vi "get.Bytes.vi"(8 "error in (no error)":errorcluster, 11 "SequencedUnitHeader in":refnum<class "SequencedUnitHeader.lvclass">) -> (0 "error out":errorcluster, 2 "Bytes.Out":u8[](array[numeric]), 3 "SequencedUnitHeader out":refnum<class "SequencedUnitHeader.lvclass">)   [LabVIEW 2020, in "SequencedUnitHeader.lvclass"]
uses:
  SequencedUnitHeader.lvclass
  SequencedUnitHeader.lvclass/SequencedUnitHeader.ctl
  MessageBase/MessageBase.lvclass
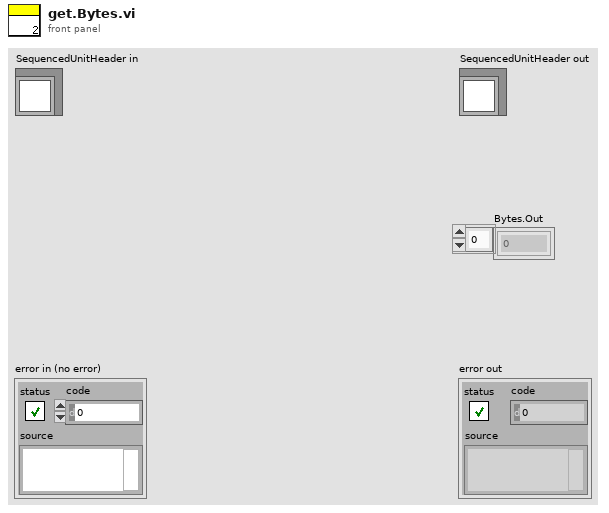
[diagram p1: front panel]
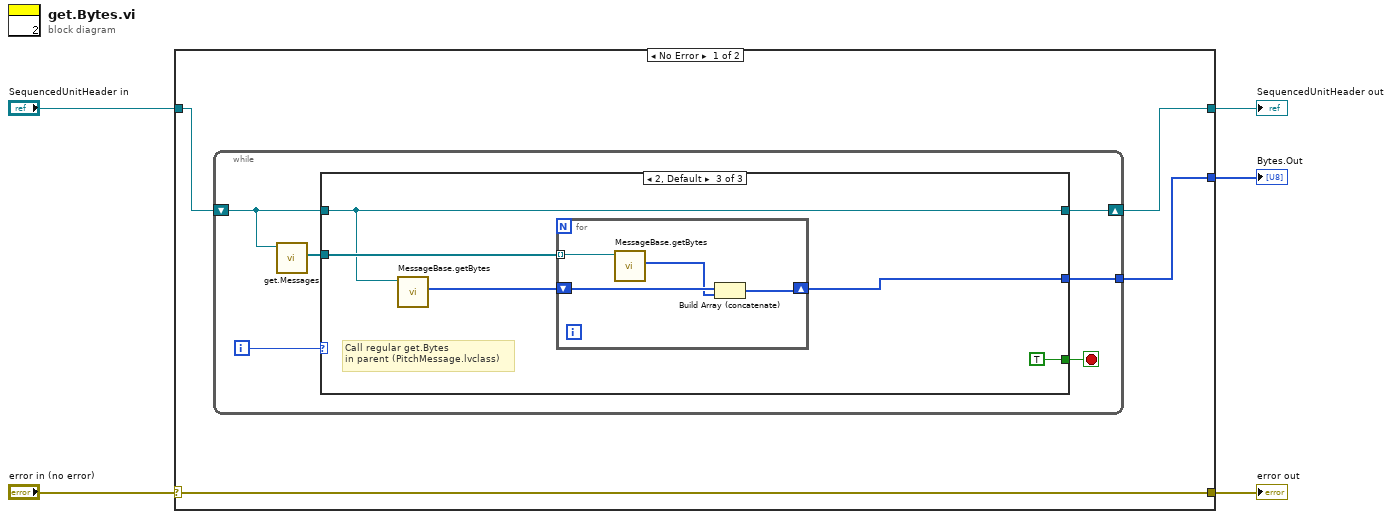
[diagram p0: block diagram]
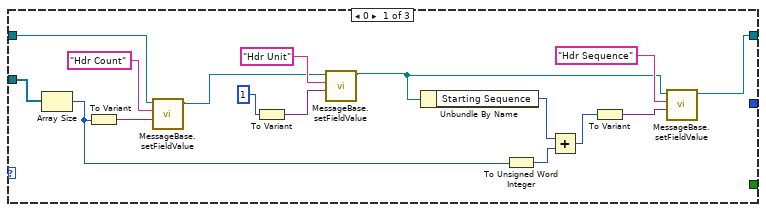
[diagram p2: hidden frame]
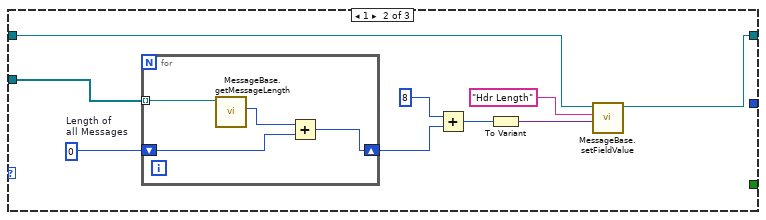
[diagram p3: hidden frame]
diagram:
  n1 = case shown="No Error" "error in (no error)" {
    selector: "error in (no error)" -> [w9 w55]
    tunnel: [w9 w55] -> w4
    tunnel: [w8 w54] -> w2
    tunnel: "SequencedUnitHeader in" -> [w6 w54]
    tunnel: [w7 _] -> w1
    frame No Error {
      n2 = while {
        shift-right: [w10] -> w8
        shift-left: w6 -> [w13]
        tunnel: [w11] -> w7
        i -> [w15]
        stop <- w14 stop-if-true
        n3 = call-dynamic "get.Messages.vi"("SequencedUnitHeader in"=w13) -> ("Messages.Out"=w12:refnum<class "MessageBase.lvclass">[])  [unwired: 8 in, 2 out]
        n4 = case shown="2, Default" w15 {
          tunnel: [_ _ TRUE] -> w14
          tunnel: w13 -> [w23 w35 w46]
          tunnel: [w18 w33 w46] -> w10
          tunnel: w12 -> [w31 w40 w48]
          tunnel: [_ _ w47] -> w11
          frame 0 {
            n5 = Array Size(array=w31) -> (size(s)=w29:i32)
            n6 = To Variant(anything=w29) -> (Variant=w25:variant)
            n7 = call-dynamic "MessageBase.setFieldValue.vi"("Value"=w25, "FIeld.Name"="Hdr Count", "MessageBase in"=w23) -> ("MessageBase out"=w20:refnum<class "SequencedUnitHeader.lvclass">)  [unwired: 7 in, 1 out]
            n8 = To Variant(anything=1) -> (Variant=w22:variant)
            n9 = call-dynamic "MessageBase.setFieldValue.vi"("Value"=w22, "FIeld.Name"="Hdr Unit", "MessageBase in"=w20) -> ("MessageBase out"=w16:refnum<class "SequencedUnitHeader.lvclass">)  [unwired: 7 in, 1 out]
            n10 = Unbundle By Name(w16) -> ("Starting Sequence"=w28:u32)
            n11 = To Unsigned Word Integer(number=w29) -> (unsigned 16bit integer=w26:u16)
            n12 = Add(x=w28, y=w26) -> (x+y=w27:u32)
            n13 = To Variant(anything=w27) -> (Variant=w17:variant)
            n14 = call-dynamic "MessageBase.setFieldValue.vi"("Value"=w17, "FIeld.Name"="Hdr Sequence", "MessageBase in"=w16) -> ("MessageBase out"=w18:refnum<class "SequencedUnitHeader.lvclass">)  [unwired: 7 in, 1 out]
          }
          frame 1 {
            w39 = u16 0  # Length of all Messages
            n15 = for {
              tunnel: w40 -> [w42] mode=indexing
              shift-right: [w43] -> w38
              shift-left: w39 -> [w44]
              n16 = call-dynamic "MessageBase.getMessageLength.vi"("MessageBase in"=w42) -> ("Length"=w41:u8)  [unwired: 8 in, 2 out]
              n17 = Add(x=w41, y=w44) -> (x+y=w43:u16)
            }
            n18 = Add(x=u16 8, y=w38) -> (x+y=w36:u16)
            n19 = To Variant(anything=w36) -> (Variant=w32:variant)
            n20 = call-dynamic "MessageBase.setFieldValue.vi"("Value"=w32, "FIeld.Name"="Hdr Length", "MessageBase in"=w35) -> ("MessageBase out"=w33:refnum<class "SequencedUnitHeader.lvclass">)  [unwired: 7 in, 1 out]
          }
          frame 2, Default {
            # "Call regular get.Bytes\nin parent (PitchMessage.lvclass)"
            n21 = call-dynamic "MessageBase.getBytes.vi"("MessageBase in"=w46) -> ("Bytes.out"=w45:u8[])  [unwired: 8 in, 2 out]
            n22 = for {
              tunnel: w48 -> [w51] mode=indexing
              shift-right: [w52] -> w47
              shift-left: w45 -> [w53]
              n23 = call-dynamic "MessageBase.getBytes.vi"("MessageBase in"=w51) -> ("Bytes.out"=w50:u8[])  [unwired: 8 in, 2 out]
              n24 = Build Array (concatenate)(w53, w50) -> (w52:u8[])
            }
          }
        }
      }
    }
    frame Error {
    }
  }
  "error out" <- w4
  "SequencedUnitHeader out" <- w2
  "Bytes.Out" <- w1
